vi "FourFlippingCoins.vi"() -> ()   [LabVIEW 2014]
panel:
  out "Number of Heads":dbl[](array[numeric])
  in  "Number of Trials":dbl
  out "Coin 4":bool
  out "Coin 3":bool
  out "Coin 2":bool
  out "Coin 1":bool
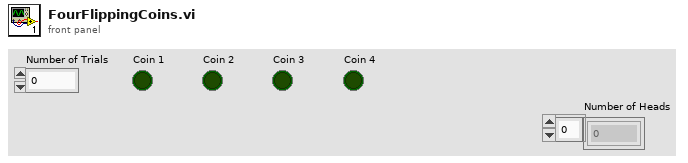
[diagram p1: front panel]
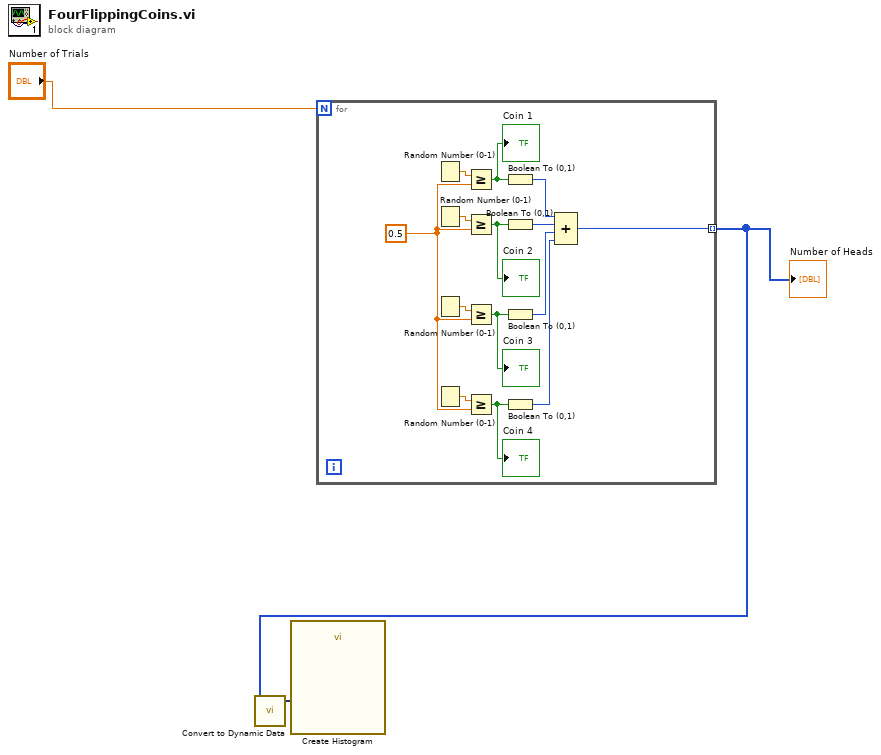
[diagram p0: block diagram]
diagram:
  n1 = for {
    N: "Number of Trials" -> [_]
    tunnel: [w4] -> w2 mode=indexing
    w13 = 0.5
    n2 = Random Number (0-1)() -> (number: 0 to 1=w9:dbl)
    n3 = Random Number (0-1)() -> (number: 0 to 1=w10:dbl)
    n4 = Random Number (0-1)() -> (number: 0 to 1=w11:dbl)
    n5 = Random Number (0-1)() -> (number: 0 to 1=w12:dbl)
    n6 = Greater Or Equal?(x=w9, y=w13) -> (x >= y?=w14:bool)
    "Coin 1" <- w14
    n7 = Greater Or Equal?(x=w10, y=w13) -> (x >= y?=w15:bool)
    "Coin 2" <- w15
    n8 = Greater Or Equal?(x=w11, y=w13) -> (x >= y?=w16:bool)
    "Coin 3" <- w16
    n9 = Greater Or Equal?(x=w12, y=w13) -> (x >= y?=w17:bool)
    "Coin 4" <- w17
    n10 = Boolean To (0,1)(Boolean=w14) -> (0, 1=w5:i16)
    n11 = Boolean To (0,1)(Boolean=w15) -> (0, 1=w6:i16)
    n12 = Boolean To (0,1)(Boolean=w16) -> (0, 1=w7:i16)
    n13 = Boolean To (0,1)(Boolean=w17) -> (0, 1=w8:i16)
    n14 = Compound Arithmetic op=ADD(w5, w6, w7, w8) -> (w4:i16)
  }
  "Number of Heads" <- w2
  n15 = call "Convert to Dynamic Data"("Array"=w2) -> ("Dynamic Data Type"=w1:dynamicdata)  [unwired: 3 in]
  n16 = call "Create Histogram"("Signal"=w1) -> ()  [unwired: 9 in, 2 out]
